vi "数据查询.vi"() -> ()   [LabVIEW 2016, in "数据查询.lvlib"]
uses:
  <vilib>/Utility/sysdir.llb/System Directory Type.ctl
  <vilib>/Utility/miscctls.llb/LVPointTypeDef.ctl
  var/holding var.vi
  <vilib>/ptbypt/NI_PtbyPt.lvlib
panel:
  out "布尔":bool
  in  "设置按钮":bool
  in  "标识说明":bool
  in  "数据查询菜单":T1
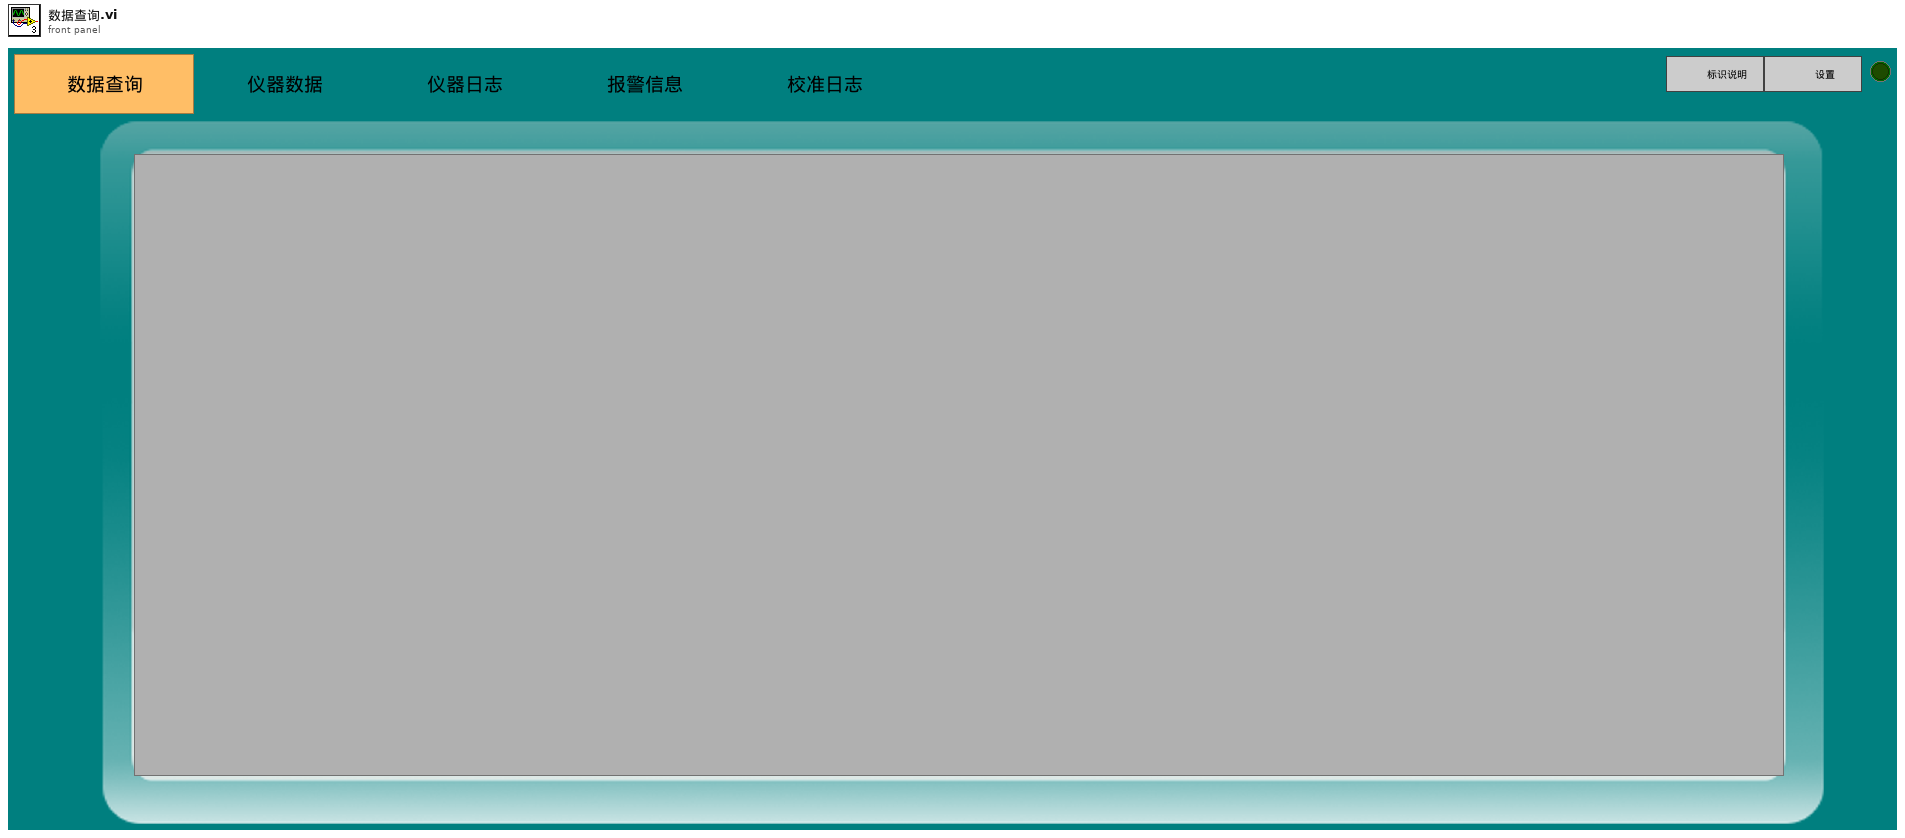
[diagram p1: front panel]
types:
  T1 = typedef "数据查询.lvlib/数据查询单选控件.ctl" = enum32{"数据查询", "仪器数据", "仪器日志", "报警信息", "校准日志"}
  T2 = typedef "LVPointTypeDef.ctl" = cluster{"Horizontal":i16, "Vertical":i16}
  T3 = typedef "LVDateTimeRec.ctl" = cluster{"秒数的小数部分":dbl, "秒":i32, "分":i32, "时":i32, "日":i32, "月":i32, "年":i32, "天数（周）":i32, "天数（年）":i32, "DST":i32}
  T4 = typedef "System Directory Type.ctl" = i32
  T5 = enum32{"Bad", "Idle", "Run top level", "Running"}
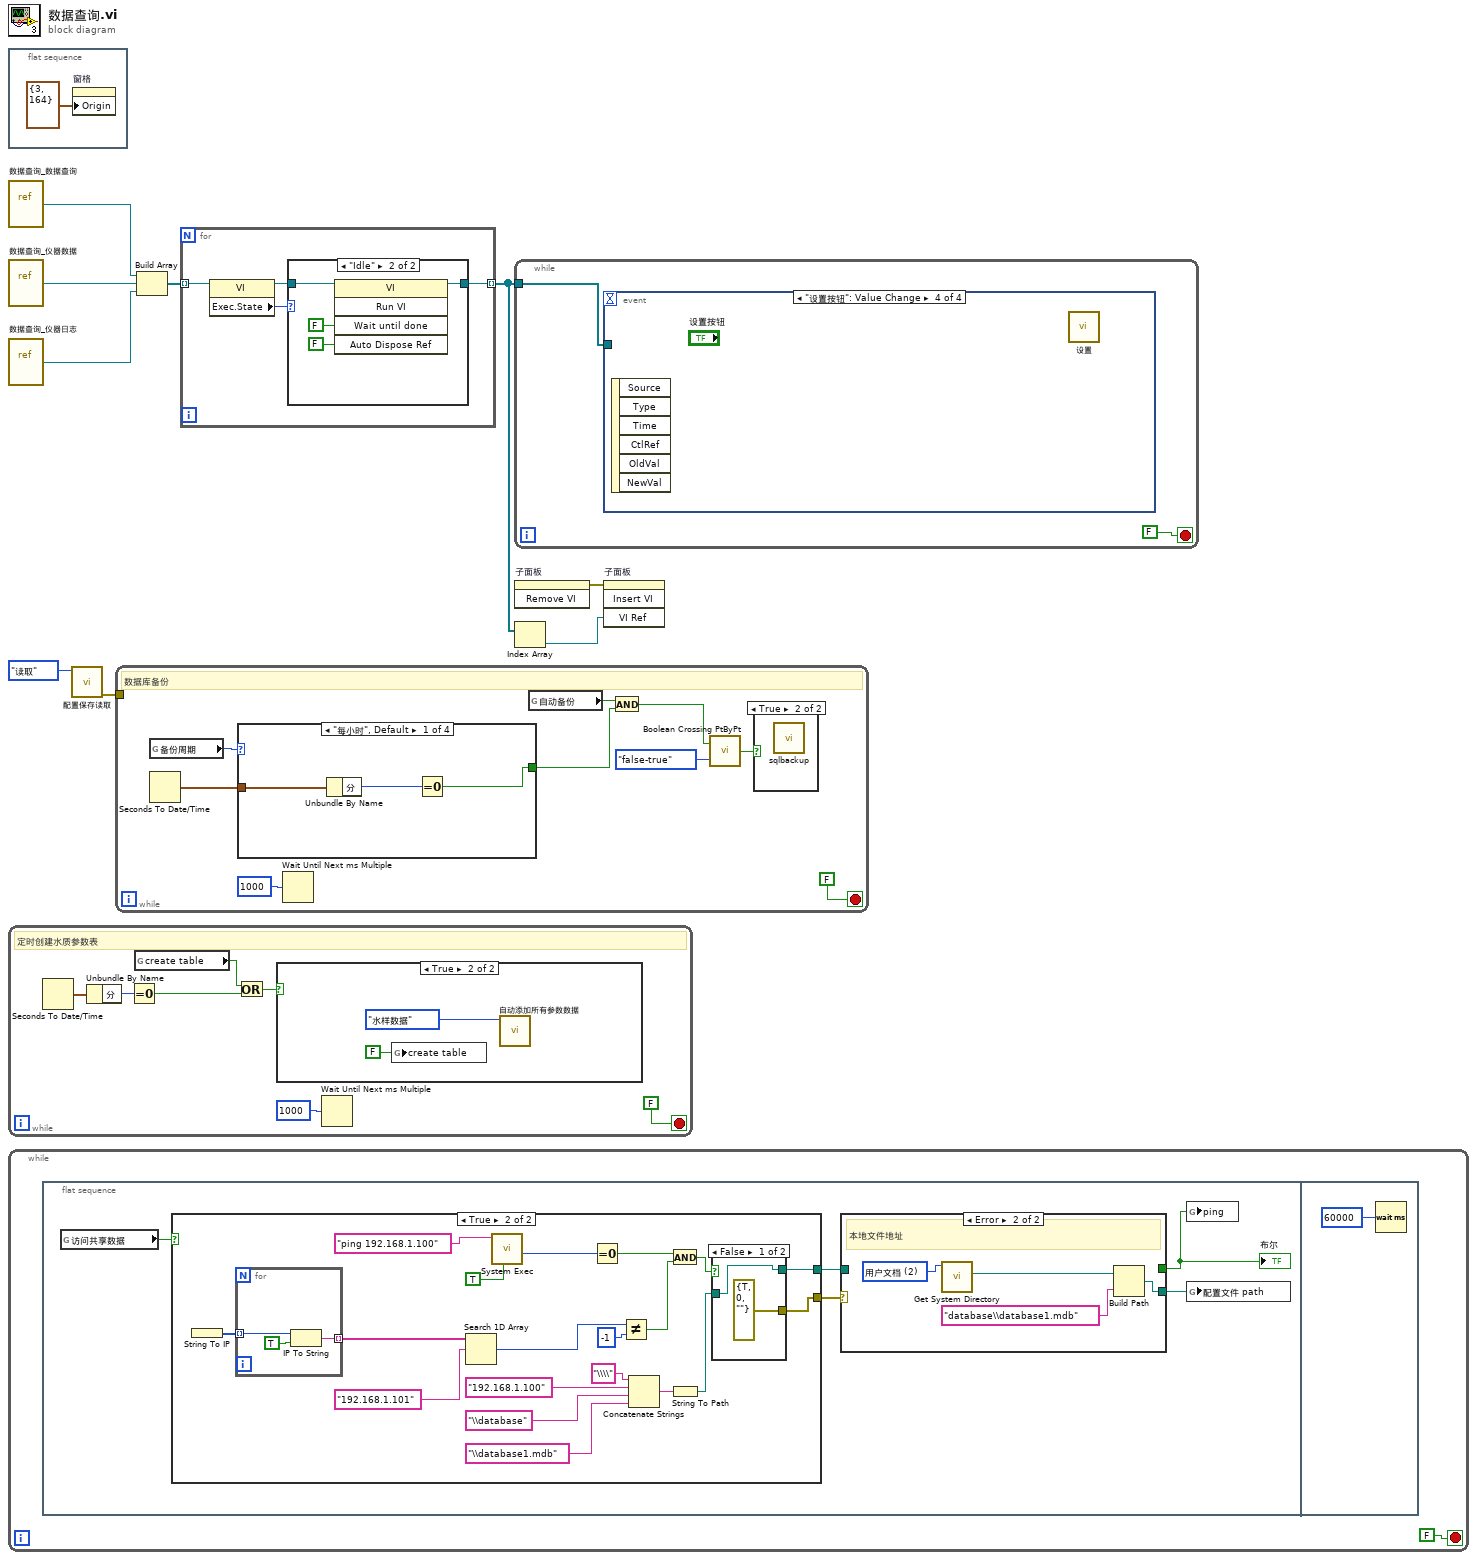
[diagram p0: block diagram]
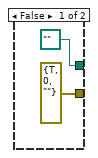
[diagram p2: hidden frame]
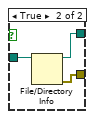
[diagram p3: hidden frame]
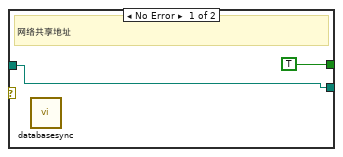
[diagram p4: hidden frame]
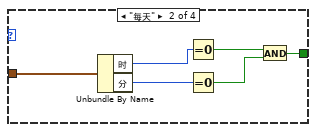
[diagram p6: hidden frame]
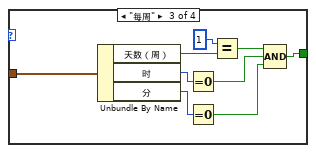
[diagram p7: hidden frame]
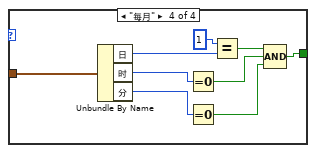
[diagram p8: hidden frame]
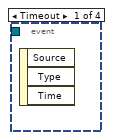
[diagram p11: hidden frame]
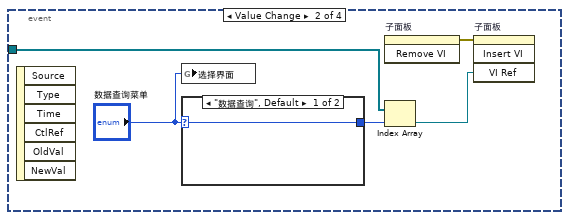
[diagram p12: hidden frame]
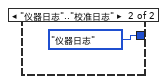
[diagram p13: hidden frame]
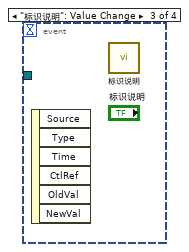
[diagram p14: hidden frame]
diagram:
  n1 = flat-sequence {
    frame #0 {
      n2 = property on="窗格" class="Pane"("Origin"=T2 {"Horizontal"=3, "Vertical"=164} ("原点")) -> ()  [unwired: 2 in, 2 out]
    }
  }
  n3 = vi-ref "数据查询_数据查询.vi"() -> (w6:refnum<vi>)
  n4 = vi-ref "数据查询_仪器数据.vi"() -> (w4:refnum<vi>)
  n5 = vi-ref "数据查询_仪器日志.vi"() -> (w3:refnum<vi>)
  n6 = while {
    stop <- FALSE stop-if-true
    # "定时创建水质参数表"
    n7 = Seconds To Date/Time() -> (date time rec=w17:T3)  [unwired: 2 in]
    n8 = Unbundle By Name(w17) -> ("分"=w16:i32)
    n9 = Equal To 0?(x=w16) -> (x = 0?=w13:bool)
    n10 = global read "全局变量.vi" "create table"() -> (w12:bool)
    n11 = Or(x=w12, y=w13) -> (x .or. y?=w14:bool)
    n12 = case shown="True" w14 {
      frame False {
      }
      frame True {
        n13 = global write "全局变量.vi" "create table"(FALSE ("create table")) -> ()
        n14 = call "自动添加所有参数数据.vi"("数据类别"=enum16{"水样数据", "日质控数据"}."水样数据") -> ()  [unwired: 10 in, 1 out]
      }
    }
    n15 = Wait Until Next ms Multiple(millisecond multiple=u32 1000 ("毫秒倍数")) -> ()  [unwired: 1 out]
  }
  n16 = while {
    stop <- FALSE stop-if-true
    n17 = flat-sequence {
      frame #0 {
        n18 = global read "全局变量.vi" "访问共享数据"() -> (w22:bool)
        n19 = case shown="True" w22 {
          tunnel: [path "" ("dup path") w40] -> w25
          tunnel: [errorcluster {"status"=TRUE, "code"=0, "source"=""} ("error out") w39] -> w24
          frame False {
          }
          frame True {
            n20 = String To IP() -> (0:w33:u32[])  [unwired: 1 in]
            n21 = for {
              tunnel: w33 -> [w49] mode=indexing
              tunnel: [w48] -> w32 mode=indexing
              n22 = IP To String(1:TRUE ("句点符号？(F)"), 2:w49) -> (0:w48:string)
            }
            n23 = Search 1D Array(1D array=w32, element="192.168.1.101" ("command line")) -> (index of element=w30:i32)  [unwired: 1 in]
            n24 = call <vilib>:"System Exec.vi"("run minimized? (F)"=TRUE, "command line"="ping 192.168.1.100") -> ("return code"=w36:i32)  [unwired: 6 in, 3 out]
            n25 = Equal To 0?(x=w36) -> (x = 0?=w35:bool)
            n26 = Not Equal?(x=w30, y=-1) -> (x != y?=w28:bool)
            n27 = Concatenate Strings("\\\\" ("字符串"), "192.168.1.100" ("名称"), "\\database" ("字符串"), "\\database1.mdb" ("名称或相对路径")) -> (w45:string)
            n28 = And(x=w35, y=w28) -> (x .and. y?=w34:bool)
            n29 = String To Path(string=w45) -> (path=w42:path)
            n30 = case shown="False" w34 {
              tunnel: w42 -> [w51 w54]
              tunnel: [w51 w53] -> w40
              tunnel: [errorcluster {"status"=TRUE, "code"=0, "source"=""} ("error out") w52] -> w39
              frame False {
              }
              frame True {
                n31 = File/Directory Info(path=w54) -> (path out=w53:path, error out=w52:errorcluster)  [unwired: 1 in, 5 out]
              }
            }
          }
        }
        n32 = case shown="Error" w24 {
          tunnel: w25 -> [w56 _]
          tunnel: [w56 w59] -> w23
          tunnel: [TRUE _] -> w21
          frame No Error {
            # "网络共享地址"
            n33 = call "databasesync.vi"() -> ()  [unwired: 12 in]
          }
          frame Error {
            w57 = T4 2 items=["用户目录"=0, "用户桌面"=1, "用户文档"=2, "用户应用程序数据"=3, "用户设置"=4, "用户临时目录"=5, "公共文档"=6, "公共应用程序数据"=7, "公共设置"=8, "公共缓存"=13, "系统核心库"=9, "系统安装库"=10, "应用程序文件"=11, "启动盘根目录"=12] ("system directory type")
            # "本地文件地址"
            n34 = call <vilib>:"Get System Directory.vi"("system directory type"=w57) -> ("system directory"=w58:path)  [unwired: 10 in]
            n35 = Build Path(base path=w58, name or relative path="database\\database1.mdb" ("名称或相对路径")) -> (appended path=w59:path)
          }
        }
        "布尔" <- w21
        n36 = global write "全局变量.vi" "ping"(w21) -> ()
        n37 = global write "全局变量.vi" "配置文件 path"(w23) -> ()
      }
      frame #1 {
        n38 = Wait (ms)(milliseconds to wait=u32 60000 ("等待时间（毫秒）")) -> ()  [unwired: 1 out]
      }
    }
  }
  n39 = call "配置保存读取.vi"("配置"=enum16{"读取", "写入"}."读取") -> ("error out"=w1:errorcluster)  [unwired: 10 in]
  n40 = while {
    tunnel: w1 -> [_]
    stop <- FALSE stop-if-true
    # "数据库备份"
    n41 = global read "holding var.vi" "备份周期"() -> (w69:enum16{"每小时", "每天", "每周", "每月"})
    n42 = Seconds To Date/Time() -> (date time rec=w64:T3)  [unwired: 2 in]
    n43 = case shown="\"每小时\", Default" w69 {
      tunnel: w64 -> [w73 w79 w88 w97]
      tunnel: [w71 w74 w80 w89] -> w63
      frame "每小时", Default {
        n44 = Unbundle By Name(w73) -> ("分"=w72:i32)
        n45 = Equal To 0?(x=w72) -> (x = 0?=w71:bool)
      }
      frame "每天" {
        n46 = Unbundle By Name(w79) -> ("时"=w77:i32, "分"=w78:i32)
        n47 = Equal To 0?(x=w77) -> (x = 0?=w75:bool)
        n48 = Equal To 0?(x=w78) -> (x = 0?=w76:bool)
        n49 = And(x=w75, y=w76) -> (x .and. y?=w74:bool)
      }
      frame "每周" {
        n50 = Unbundle By Name(w88) -> ("天数（周）"=w87:i32, "时"=w85:i32, "分"=w84:i32)
        n51 = Equal To 0?(x=w85) -> (x = 0?=w82:bool)
        n52 = Equal To 0?(x=w84) -> (x = 0?=w81:bool)
        n53 = Equal?(x=1, y=w87) -> (x = y?=w83:bool)
        n54 = Compound Arithmetic op=AND ("复合运算")(w83, w82, w81) -> (w80:bool)
      }
      frame "每月" {
        n55 = Unbundle By Name(w97) -> ("日"=w96:i32, "时"=w94:i32, "分"=w93:i32)
        n56 = Equal To 0?(x=w94) -> (x = 0?=w91:bool)
        n57 = Equal To 0?(x=w93) -> (x = 0?=w90:bool)
        n58 = Equal?(x=1, y=w96) -> (x = y?=w92:bool)
        n59 = Compound Arithmetic op=AND ("复合运算")(w92, w91, w90) -> (w89:bool)
      }
    }
    n60 = Wait Until Next ms Multiple(millisecond multiple=u32 1000 ("毫秒倍数")) -> ()  [unwired: 1 out]
    n61 = global read "holding var.vi" "自动备份"() -> (w68:bool)
    n62 = And(x=w68, y=w63) -> (x .and. y?=w67:bool)
    n63 = call <vilib>:"Boolean Crossing PtByPt.vi"("direction"=enum16{"either", "false-true", "true-false"}."false-true", "input"=w67) -> ("crossing"=w65:bool)  [unwired: 1 in]
    n64 = case shown="True" w65 {
      frame False {
      }
      frame True {
        n65 = call "sqlbackup.vi"() -> ()  [unwired: 11 in, 1 out]
      }
    }
  }
  n66 = Build Array(w6, w4, w3) -> (w5:refnum<vi>[])
  n67 = for {
    tunnel: w5 -> [w101] mode=indexing
    tunnel: [w98] -> w8 mode=indexing
    n68 = property class="VI"(reference=w101) -> (reference out=w99:refnum<vi>, "Exec.State"=w100:T5)  [unwired: 1 in, 1 out]
    n69 = case shown="\"Idle\"" w100 {
      tunnel: w99 -> [w102 w104]
      tunnel: [w102 w103] -> w98
      frame "Bad", Default {
      }
      frame "Idle" {
        n70 = invoke class="VI" method="Run VI"(reference=w104, "Wait until done"=FALSE ("结束前等待"), "Auto Dispose Ref"=FALSE ("自动销毁引用")) -> (reference out=w103:refnum<vi>)  [unwired: 2 in, 4 out]
      }
    }
  }
  n71 = while {
    tunnel: w8 -> [w107]
    stop <- FALSE stop-if-true
    n72 = event shown="[3] \"设置按钮\": Value Change" {
      selector: _ -> [_ _ _ _]
      dyn-events: _ -> [_ _ _ _]
      timeout: _ -> [_ _ _ _]
      tunnel: w107 -> [_ w113 _ _]
      event Timeout {
        n73 = event-data() -> ()  [unwired: 1 in, 3 out]
      }
      event Value Change {
        n74 = event-data() -> ()  [unwired: 1 in, 6 out]
        n75 = global write "全局变量.vi" "选择界面"("数据查询菜单") -> ()
        n76 = case shown="\"数据查询\", Default" "数据查询菜单" {
          selector: "数据查询菜单" -> [w114 _]
          tunnel: [w114 enum32{"数据查询", "仪器数据", "仪器日志", "报警信息", "校准日志"}."仪器日志" ("数据查询菜单")] -> w110
          frame "数据查询", Default {
          }
          frame "仪器日志".."校准日志" {
          }
        }
        n77 = invoke on="子面板" class="SubPnl" method="Remove VI"() -> (error out=w111:errorcluster)  [unwired: 3 in, 2 out]
        n78 = Index Array(array=w113, index=w110) -> (element=w112:refnum<vi>)
        n79 = invoke on="子面板" class="SubPnl" method="Insert VI"(error in=w111, "VI Ref"=w112) -> ()  [unwired: 2 in, 4 out]
      }
      event "标识说明": Value Change {
        n80 = event-data() -> ()  [unwired: 1 in, 6 out]
        n81 = call "标识说明.vi"() -> ()  [unwired: 12 in]
      }
      event "设置按钮": Value Change {
        n82 = event-data() -> ()  [unwired: 1 in, 6 out]
        n83 = call "设置.vi"() -> ()  [unwired: 12 in]
      }
    }
  }
  n84 = invoke on="子面板" class="SubPnl" method="Remove VI"() -> (error out=w9:errorcluster)  [unwired: 3 in, 2 out]
  n85 = Index Array(array=w8) -> (element=w7:refnum<vi>)  [unwired: 1 in]
  n86 = invoke on="子面板" class="SubPnl" method="Insert VI"(error in=w9, "VI Ref"=w7) -> ()  [unwired: 2 in, 4 out]
